vi "Center in Subdiagram.vi"(6 "Variant in":variant, 7 "Shift Pressed?":bool, 8 "error in (no error)":errorcluster, 10 "QD Combo Box Ref":refnum<vi>, 11 "QD Launch VI Ref":refnum<vi>) -> (0 "error out":errorcluster, 4 "Variant out":variant)   [LabVIEW 2017]
doc: "Write a 1-2 sentence description of the functionality of your plugin here. Replace the \"$\" below with the character you wish to assign as the default shortcut for this plugin. Do not add any text after the 'Default Shortcut' line below.\n\nDefault Shortcut - [$]"
panel:
  in  "Undo Name":string="Quick Drop Keyboard Shortcut"
  # "Do not change the connector pane of this VI.\n\nSee the block diagram for directions on how to use this template."
  # "Specify the name of the Undo transaction"
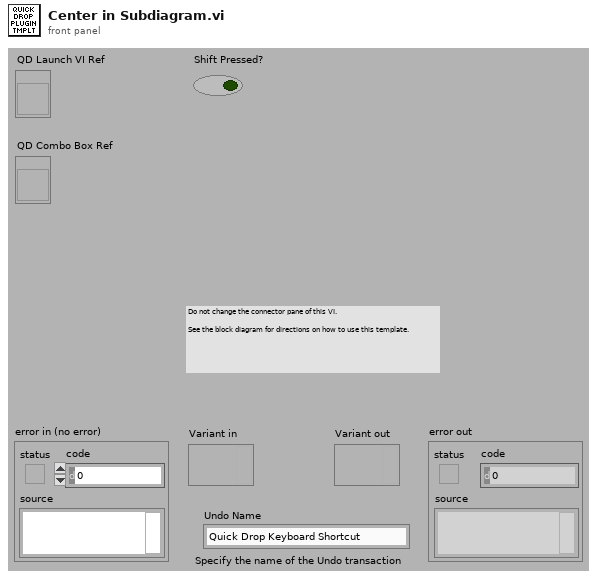
[diagram p1: front panel]
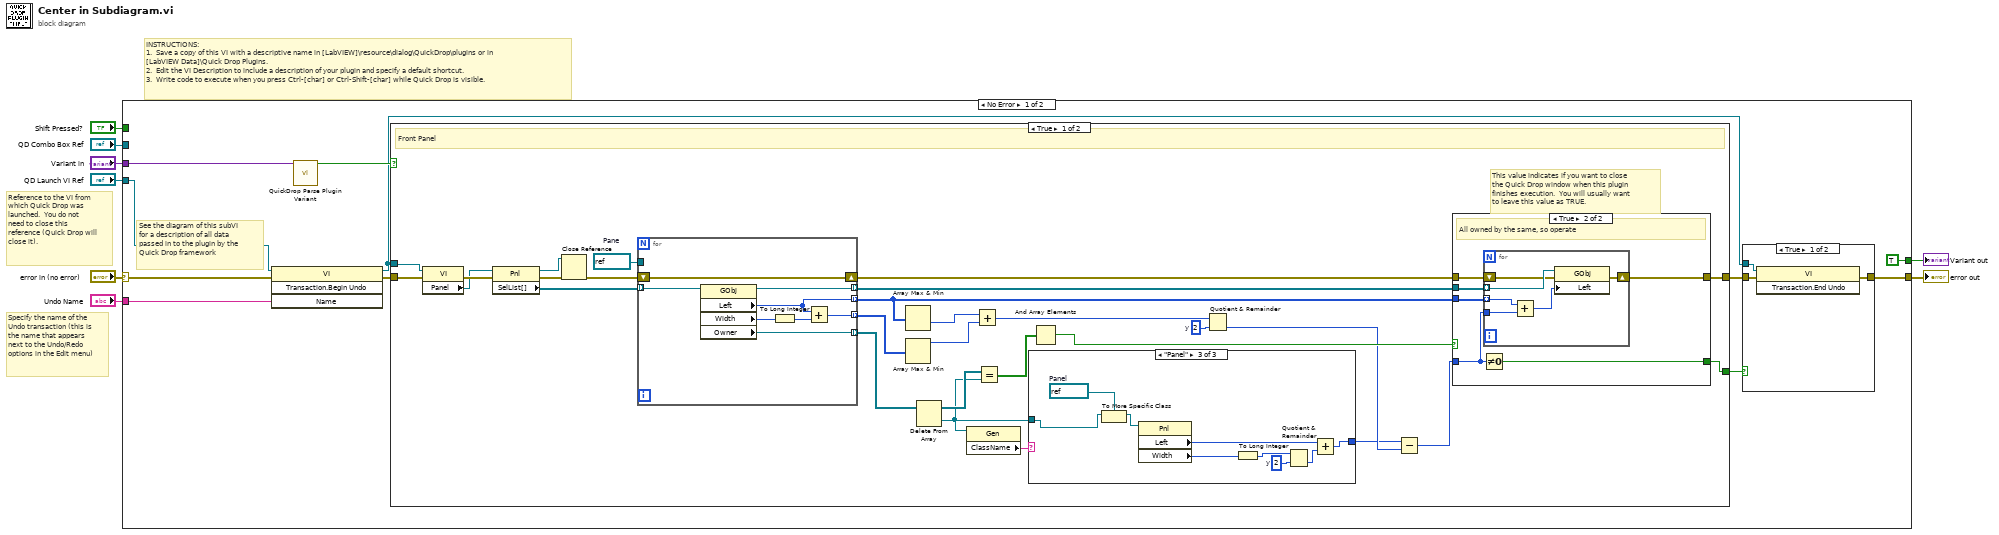
[diagram p0: block diagram]
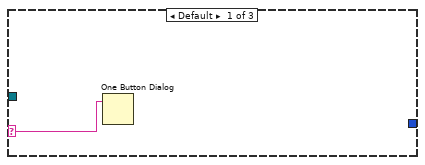
[diagram p2: hidden frame]
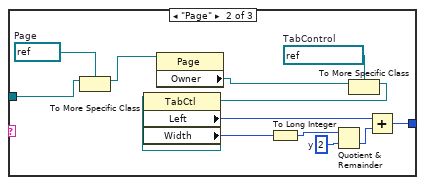
[diagram p3: hidden frame]
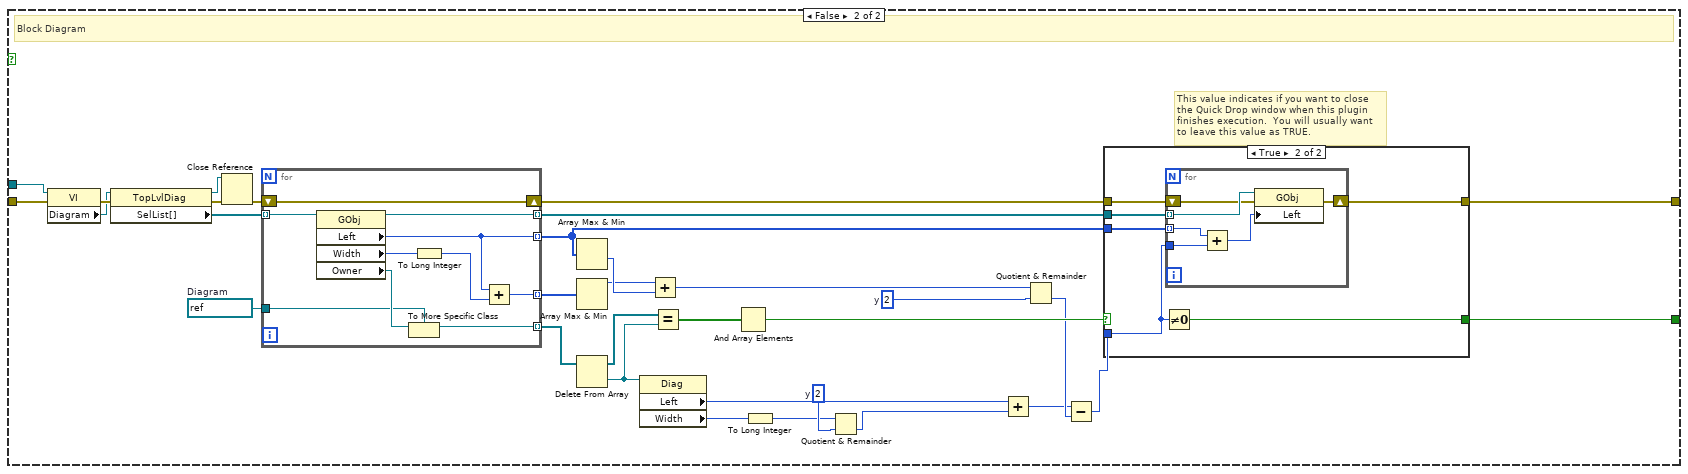
[diagram p5: hidden frame]
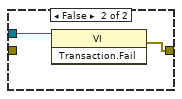
[diagram p7: hidden frame]
diagram:
  # "Specify the name of the Undo transaction (this is the name that appears next to the Undo/Redo options in the Edit menu)"
  # "Reference to the VI from which Quick Drop was launched.  You do not need to close this reference (Quick Drop will close it)."
  # "INSTRUCTIONS:\n1.  Save a copy of this VI with a descriptive name in [LabVIEW]\\resource\\dialog\\QuickDrop\\plugins or in [LabVIEW Data]\\Quick Drop Plugins.\n2.  Edit the VI Description to include a description of your plugin and specify a default shortcut. \n3.  Write code to execute when you press Ctrl-[char] or Ctrl-Shift-[char] while Quick Drop is visible."
  n1 = case shown="No Error" "error in (no error)" {
    selector: "error in (no error)" -> [w18 w153]
    tunnel: [w12 w153] -> w7
    tunnel: "QD Launch VI Ref" -> [w17 _]
    tunnel: "Shift Pressed?" -> [_ _]
    tunnel: "QD Combo Box Ref" -> [_ _]
    tunnel: "Variant in" -> [w19 _]
    tunnel: "Undo Name" -> [w16 _]
    tunnel: [TRUE _] -> w1
    frame No Error {
      # "See the diagram of this subVI for a description of all data passed in to the plugin by the Quick Drop framework"
      n2 = invoke class="VI" method="Transaction.Begin Undo"(reference=w17, error in=w18, "Name"=w16) -> (reference out=w11:refnum<vi>, error out=w13:errorcluster)  [unwired: 1 in, 2 out]
      n3 = call <vilib>:"QuickDrop Parse Plugin Variant.vi"("QDKS Variant in"=w19) -> ("QD Launch VI Panel?"=w14:bool)  [unwired: 12 in, 2 out]
      n4 = case shown="True" w14 {
        tunnel: w13 -> [w47 w123]
        tunnel: w11 -> [w45 w121]
        tunnel: [w36 w107] -> w10
        tunnel: [w34 w105] -> w9
        frame True {
          w26 = refnum<vi> refnum  # Pane
          w33 = 2  # y
          # "This value indicates if you want to close the Quick Drop window when this plugin finishes execution.  You will usually want to leave this value as TRUE."
          # "Front Panel"
          n5 = property class="VI"(reference=w45, error in=w47) -> (error out=w25:errorcluster, "Panel"=w24:refnum<vi>)  [unwired: 1 out]
          n6 = property class="Pnl"(reference=w24, error in=w25) -> (reference out=w22:refnum<vi>, error out=w23:errorcluster, "SelList[]"=w44:refnum<vi>[])
          n7 = Close Reference(reference=w22, error in (no error)=w23) -> (error out=w46:errorcluster)
          n8 = for {
            shift-right: [w91] -> w39
            shift-left: w46 -> [w91]
            tunnel: w44 -> [w90] mode=indexing
            tunnel: [w84] -> w41 mode=indexing
            tunnel: [w89] -> w38 mode=indexing
            tunnel: [w87] -> w40 mode=indexing
            tunnel: [w86] -> w37 mode=indexing
            tunnel: w26 -> [_]
            n9 = property class="GObj"(reference=w90) -> (reference out=w89:refnum<vi>, "Left"=w86:i32, "Width"=w88:u32, "Owner"=w84:refnum<vi>)  [unwired: 1 in, 1 out]
            n10 = To Long Integer(number=w88) -> (32bit integer=w85:i32)
            n11 = Add(x=w86, y=w85) -> (x+y=w87:i32)
          }
          n12 = Array Max & Min(array=w37) -> (min value=w30:i32)  [unwired: 3 out]
          n13 = Array Max & Min(array=w40) -> (max value=w29:i32)  [unwired: 3 out]
          n14 = Delete From Array(array=w41) -> (deleted portion=w21:refnum<vi>, array with subset deleted=w43:refnum<vi>[])  [unwired: 2 in]
          n15 = property class="Gen"(reference=w21) -> ("ClassName"=w20:string)  [unwired: 1 in, 2 out]
          n16 = Add(x=w30, y=w29) -> (x+y=w32:i32)
          n17 = Equal?(x=w43, y=w21) -> (x = y?=w42:bool[])
          n18 = case shown="\"Panel\"" w20 {
            selector: w20 -> [w48 _ _]
            tunnel: [_ w56 w61] -> w28
            tunnel: w21 -> [_ w54 w68]
            frame Default {
              n19 = One Button Dialog(message=w48) -> ()  [unwired: 1 in, 1 out]
            }
            frame "Page" {
              w51 = refnum<vi> refnum  # TabControl
              w53 = refnum<vi> refnum  # Page
              w59 = 2  # y
              n20 = To More Specific Class(target class=w53, reference=w54) -> (specific class reference=w52:refnum<vi>)  [unwired: 1 in, 1 out]
              n21 = property class="Page"(reference=w52) -> ("Owner"=w50:refnum<vi>)  [unwired: 1 in, 2 out]
              n22 = To More Specific Class(target class=w51, reference=w50) -> (specific class reference=w49:refnum<vi>)  [unwired: 1 in, 1 out]
              n23 = property class="TabCtl"(reference=w49) -> ("Left"=w55:i32, "Width"=w60:u32)  [unwired: 1 in, 2 out]
              n24 = To Long Integer(number=w60) -> (32bit integer=w57:i32)
              n25 = Quotient & Remainder(x=w57, y=w59) -> (floor(x/y)=w58:i32)  [unwired: 1 out]
              n26 = Add(x=w55, y=w58) -> (x+y=w56:i32)
            }
            frame "Panel" {
              w66 = 2  # y
              w69 = refnum<vi> refnum  # Panel
              n27 = To More Specific Class(target class=w69, reference=w68) -> (specific class reference=w62:refnum<vi>)  [unwired: 1 in, 1 out]
              n28 = property class="Pnl"(reference=w62) -> ("Left"=w63:i32, "Width"=w67:u32)  [unwired: 1 in, 2 out]
              n29 = To Long Integer(number=w67) -> (32bit integer=w64:i32)
              n30 = Quotient & Remainder(x=w64, y=w66) -> (floor(x/y)=w65:i32)  [unwired: 1 out]
              n31 = Add(x=w63, y=w65) -> (x+y=w61:i32)
            }
          }
          n32 = And Array Elements(Boolean array=w42) -> (logical AND=w35:bool)
          n33 = Quotient & Remainder(x=w32, y=w33) -> (floor(x/y)=w31:i32)  [unwired: 1 out]
          n34 = Subtract(x=w28, y=w31) -> (x-y=w27:i32)
          n35 = case shown="True" w35 {
            selector: w35 -> [w71 _]
            tunnel: w39 -> [w70 w77]
            tunnel: w38 -> [_ w76]
            tunnel: w37 -> [_ w75]
            tunnel: w27 -> [_ w74]
            tunnel: [w71 w73] -> w36
            tunnel: [w70 w72] -> w34
            frame False {
            }
            frame True {
              # "All owned by the same, so operate"
              n36 = Not Equal To 0?(x=w74) -> (x != 0?=w73:bool)
              n37 = for {
                shift-right: [w81] -> w72
                shift-left: w77 -> [w82]
                tunnel: w76 -> [w83] mode=indexing
                tunnel: w75 -> [w80] mode=indexing
                tunnel: w74 -> [w79]
                n38 = Add(x=w80, y=w79) -> (x+y=w78:i32)
                n39 = property class="GObj"(reference=w83, error in=w82, "Left"=w78) -> (error out=w81:errorcluster)  [unwired: 1 out]
              }
            }
          }
        }
        frame False {
          w96 = refnum<vi> refnum  # Diagram
          w104 = 2  # y
          w113 = 2  # y
          # "This value indicates if you want to close the Quick Drop window when this plugin finishes execution.  You will usually want to leave this value as TRUE."
          # "Block Diagram"
          n40 = property class="VI"(reference=w121, error in=w123) -> (error out=w95:errorcluster, "Diagram"=w94:refnum<vi>)  [unwired: 1 out]
          n41 = property class="TopLvlDiag"(reference=w94, error in=w95) -> (reference out=w92:refnum<vi>, error out=w93:errorcluster, "SelList[]"=w120:refnum<vi>[])
          n42 = Close Reference(reference=w92, error in (no error)=w93) -> (error out=w122:errorcluster)
          n43 = for {
            shift-right: [w147] -> w111
            shift-left: w122 -> [w147]
            tunnel: w120 -> [w146] mode=indexing
            tunnel: [w144] -> w117 mode=indexing
            tunnel: [w143] -> w110 mode=indexing
            tunnel: [w141] -> w115 mode=indexing
            tunnel: [w140] -> w109 mode=indexing
            tunnel: w96 -> [w138]
            n44 = property class="GObj"(reference=w146) -> (reference out=w143:refnum<vi>, "Left"=w140:i32, "Width"=w142:u32, "Owner"=w145:refnum<vi>)  [unwired: 1 in, 1 out]
            n45 = To More Specific Class(target class=w138, reference=w145) -> (specific class reference=w144:refnum<vi>)  [unwired: 1 in, 1 out]
            n46 = To Long Integer(number=w142) -> (32bit integer=w139:i32)
            n47 = Add(x=w140, y=w139) -> (x+y=w141:i32)
          }
          n48 = Array Max & Min(array=w109) -> (min value=w101:i32)  [unwired: 3 out]
          n49 = Array Max & Min(array=w115) -> (max value=w100:i32)  [unwired: 3 out]
          n50 = Delete From Array(array=w117) -> (deleted portion=w116:refnum<vi>, array with subset deleted=w119:refnum<vi>[])  [unwired: 2 in]
          n51 = property class="Diag"(reference=w116) -> ("Left"=w98:i32, "Width"=w114:u32)  [unwired: 1 in, 2 out]
          n52 = Add(x=w100, y=w101) -> (x+y=w103:i32)
          n53 = Equal?(x=w119, y=w116) -> (x = y?=w118:bool[])
          n54 = And Array Elements(Boolean array=w118) -> (logical AND=w106:bool)
          n55 = To Long Integer(number=w114) -> (32bit integer=w108:i32)
          n56 = Quotient & Remainder(x=w108, y=w113) -> (floor(x/y)=w112:i32)  [unwired: 1 out]
          n57 = Add(x=w98, y=w112) -> (x+y=w99:i32)
          n58 = Quotient & Remainder(x=w103, y=w104) -> (floor(x/y)=w102:i32)  [unwired: 1 out]
          n59 = Subtract(x=w99, y=w102) -> (x-y=w97:i32)
          n60 = case shown="True" w106 {
            selector: w106 -> [w125 _]
            tunnel: w111 -> [w124 w131]
            tunnel: w110 -> [_ w130]
            tunnel: w109 -> [_ w129]
            tunnel: w97 -> [_ w128]
            tunnel: [w125 w127] -> w107
            tunnel: [w124 w126] -> w105
            frame False {
            }
            frame True {
              n61 = Not Equal To 0?(x=w128) -> (x != 0?=w127:bool)
              n62 = for {
                shift-right: [w135] -> w126
                shift-left: w131 -> [w136]
                tunnel: w130 -> [w137] mode=indexing
                tunnel: w129 -> [w134] mode=indexing
                tunnel: w128 -> [w133]
                n63 = Add(x=w134, y=w133) -> (x+y=w132:i32)
                n64 = property class="GObj"(reference=w137, error in=w136, "Left"=w132) -> (error out=w135:errorcluster)  [unwired: 1 out]
              }
            }
          }
        }
      }
      n65 = case shown="True" w10 {
        tunnel: w11 -> [w149 w151]
        tunnel: [w150 w152] -> w12
        tunnel: w9 -> [w148 _]
        frame True {
          n66 = invoke class="VI" method="Transaction.End Undo"(reference=w149, error in=w148) -> (error out=w150:errorcluster)  [unwired: 1 in, 2 out]
        }
        frame False {
          n67 = invoke class="VI" method="Transaction.Fail"(reference=w151) -> (error out=w152:errorcluster)  [unwired: 2 in, 2 out]
        }
      }
    }
    frame Error {
    }
  }
  "error out" <- w7
  "Variant out" <- w1
